vi "Console_Init.vi"(11 "Python":T2) -> (0 "error out":errorcluster, 1 "Console":string, 3 "Python out":T2, 5 "Disabled":T1(ring))   [LabVIEW 2022 SP3]
uses:
  PythonCtrl.ctl
  Processors.ctl
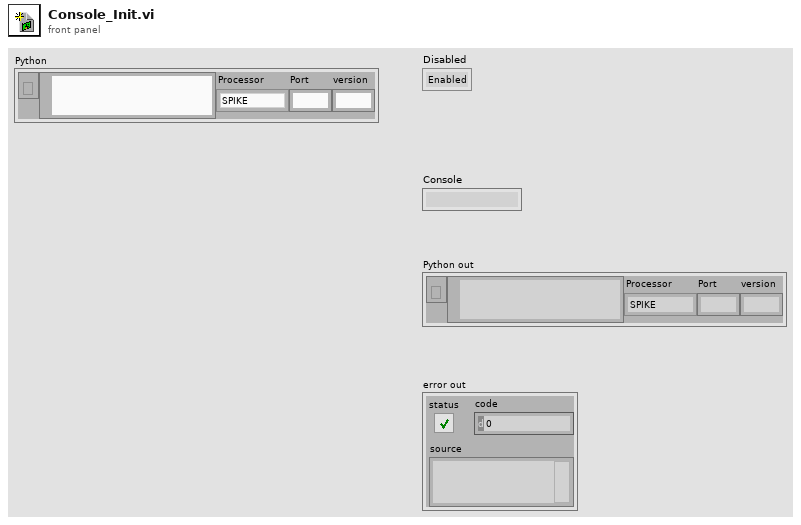
[diagram p1: front panel]
types:
  T1 = enum8{"Enabled", "Disabled", "Disabled and Grayed Out"}
  T2 = typedef "PythonCtrl.ctl" = cluster{"session":refnum<k35>, "PyPath":path, "Processor":T3, "Port":string, "version":string}
  T3 = typedef "Processors.ctl" = enum16{"SPIKE", "Pi", "Pi_ssh", "OpenMV", "Dunio"}
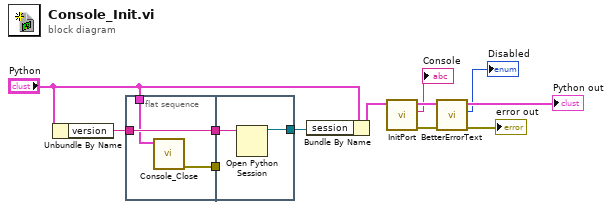
[diagram p0: block diagram]
diagram:
  n1 = Unbundle By Name("Python") -> ("version"=w3:string)
  n2 = flat-sequence {
    tunnel: [w13] -> w4
    tunnel: w3 -> [w13]
    tunnel: "Python" -> [w12]
    tunnel: [w11] -> w1
    tunnel: [w15] -> w5
    tunnel: w4 -> [w14]
    tunnel: w1 -> [_]
    frame #0 {
      n3 = call "Console_Close.vi"("Python in"=w12) -> ("error out"=w11:errorcluster)  [unwired: 10 in]
    }
    frame #1 {
      n4 = Open Python Session(python version=w14) -> (session out=w15:refnum<k35>)  [unwired: 2 in, 1 out]
    }
  }
  n5 = Bundle By Name(cluster="Python", "session"=w5) -> (w10:T2)
  n6 = call "InitPort.vi"("Python"=w10) -> ("error out"=w7:errorcluster, "Console"=→"Console":string, "Python out"=w9:T2)  [unwired: 8 in]
  "Python out" <- w9
  "error out" <- w7
  n7 = call "BetterErrorText.vi"("error in (no error)"=w7, "Python"=w9) -> ("Disabled"=→"Disabled":T1)  [unwired: 8 in, 1 out]
